vi "Read_Wavedump_Files.vi"(11 "PMTs":string[](array[string])) -> (1 "Plotted data":i32[][][](array[numeric]), 3 "Time Elapsed (s)":u32)   [LabVIEW 2018]
panel:
  in  "Test":string(combo)
  in  "Stop":bool
  in  "?":T1(tab)
  out "Waveform Graph":cluster{"Trace":i32[]}[](graph)
  in  "Viewing Rate (Trace/s)":u32=1 min=1
  in  "Start":bool
  out "Scroll Graph":i32[](graph)
  out "End of file":bool
  in  "Trace":i64
  in  "PMT Number":string
  in  "Close":bool
  # "Plotted data as 3D array"
  # "Channel"
  # "Trace"
  # "Sample"
  # "This vi is used to view previously tested PMTs at a rate of one trace per second for the length of time of recording. PMTs being tested will be viewed using the GNU plot pop up window.\n\nAuto Viewing Tab:\n\nUsed to view waveforms recorded by automattically scrolling through the data at a rate of one recorded waveform in 10000 for the 10 KHz tests (1 in 1000 for files used to develop)\n\nTo view up to 8 PMTs (one electrical tests worth), please enter the test type and the PMT numbers. Then enter the rate at which traces are viewed per second.\n\nPress \"Start\" to start viewing.\n\nUse the tick boxes to change the plots visible. The plots are in the same order the PMT numbers are entered in.\n\nPress \"STOP\" to stop viewing the files.\n\nManual Viewing Tab:\n\nUsed to manually scroll through waveforms one at a  time.\n\nEnter test and PMT number, before selecting which trace to view.\n\nA light indicates if the end of the file has been reached.\n\nPlease note, if the Auto Viewing is running, the Manual Viewing will not work. Please stop this to use the Manual Viewing tab.\n\n\n\n\nPress \"CLOSE\" to close the application."
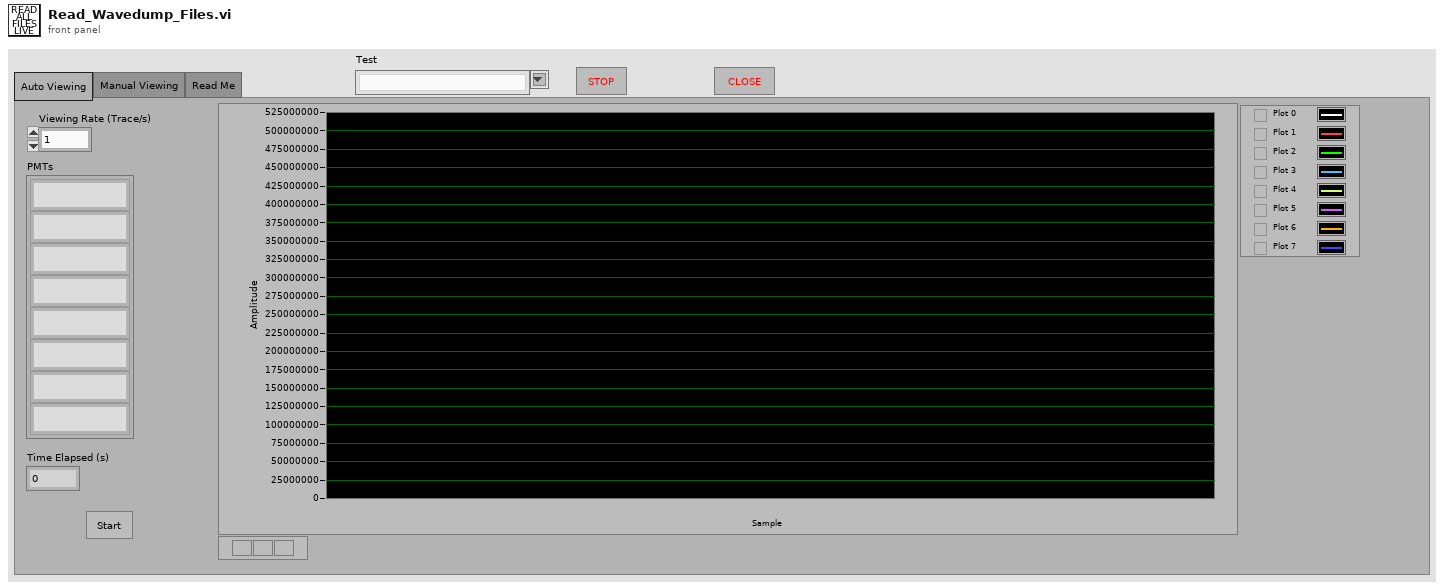
[diagram p1: front panel]
types:
  T1 = enum32{"Auto Viewing", "Manual Viewing", "Read Me"}
  T2 = enum16{"big-endian, network order", "native, host order", "little-endian"}
  T3 = enum16{"open", "replace", "create", "open or create", "replace or create", "replace or create with confirmation"}
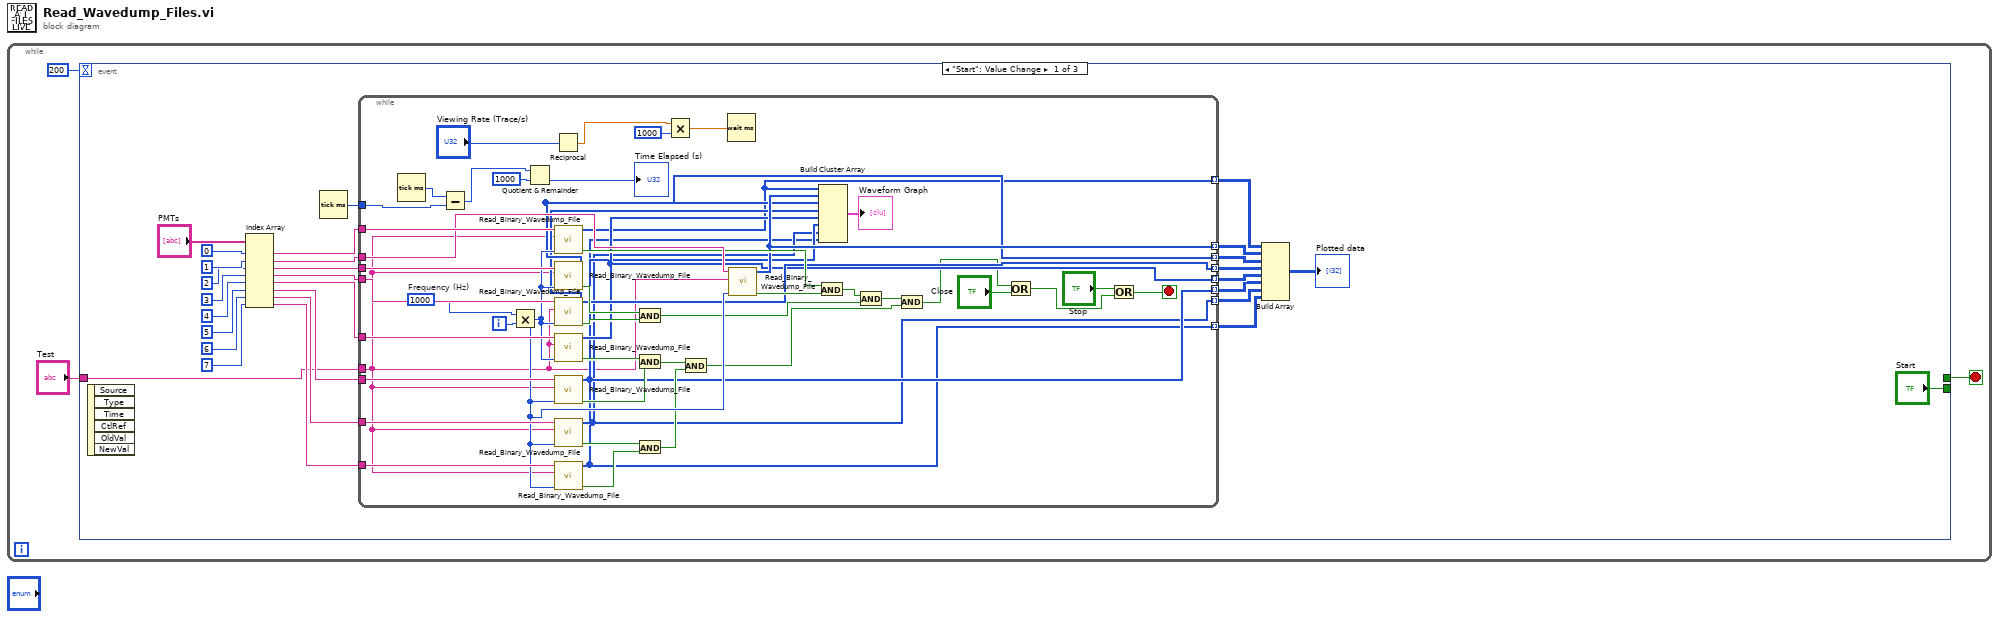
[diagram p0: block diagram]
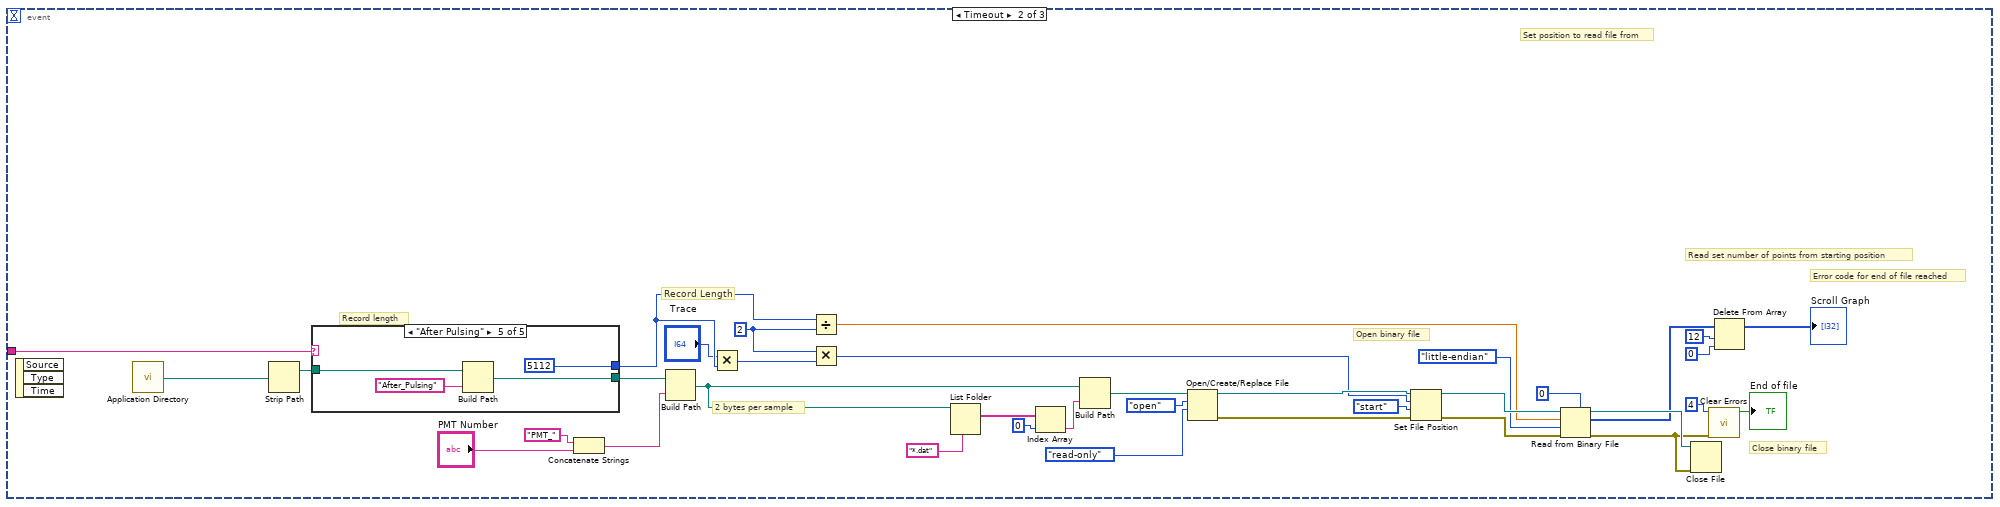
[diagram p2: hidden frame]
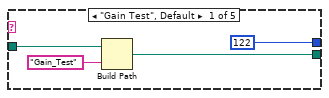
[diagram p3: hidden frame]
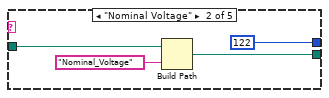
[diagram p4: hidden frame]
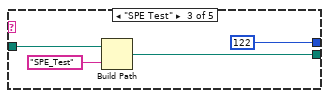
[diagram p5: hidden frame]
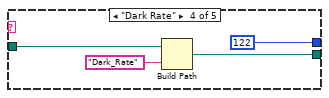
[diagram p6: hidden frame]
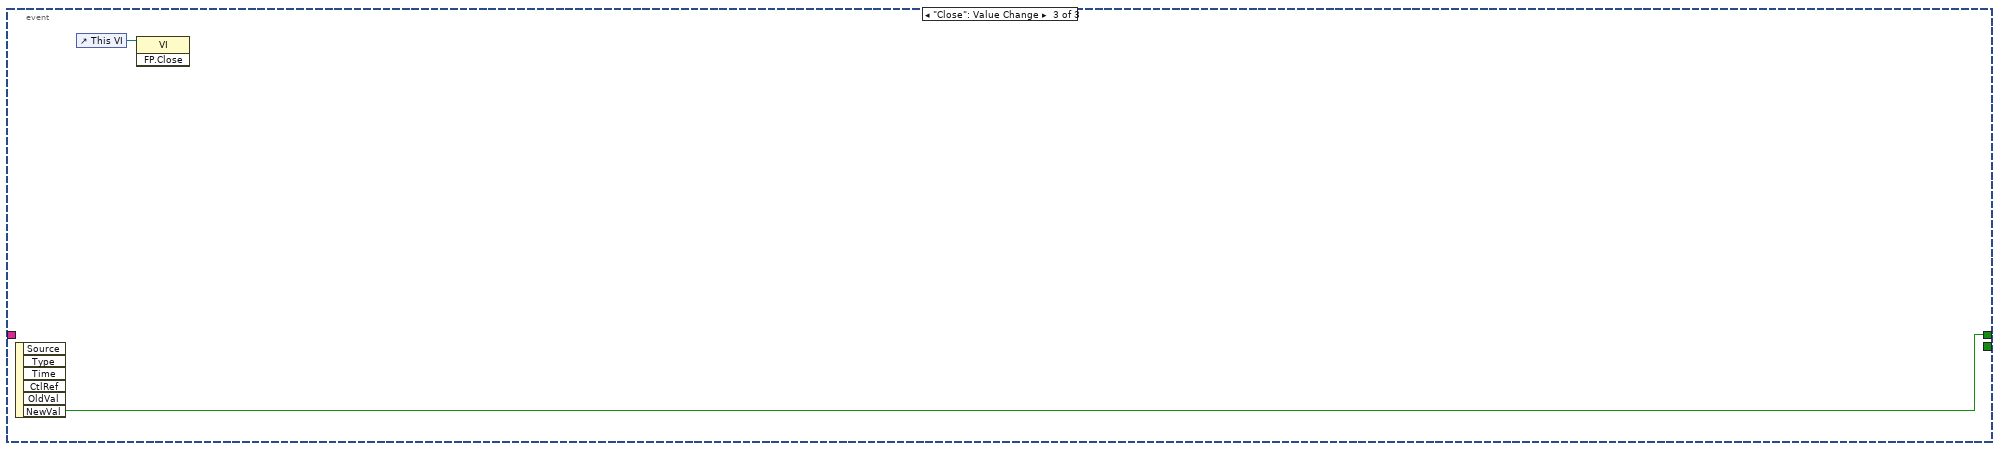
[diagram p7: hidden frame]
diagram:
  n1 = while {
    stop <- w3 stop-if-true
    n2 = event shown="[0] \"Start\": Value Change" {
      selector: _ -> [_ _ _]
      dyn-events: _ -> [_ _ _]
      timeout: 200 -> [_ _ _]
      tunnel: [_ _ w139] -> w3
      tunnel: ["Start" _ _] -> _
      tunnel: "Test" -> [w4 w83 _]
      event "Start": Value Change {
        n3 = event-data() -> ()  [unwired: 1 in, 6 out]
        n4 = Index Array(array="PMTs", index #1=0 ("index"), index #2=1 ("index"), index #3=2 ("index"), index #4=3 ("index"), index #5=4 ("index"), index #6=5 ("index"), index #7=6 ("index"), index #8=7 ("index")) -> (element #1=w24:string, element #2=w23:string, element #3=w22:string, element #4=w21:string, element #5=w20:string, element #6=w19:string, element #7=w18:string, element #8=w17:string)
        n5 = Tick Count (ms)() -> (millisecond timer value=w16:u32)
        n6 = while {
          tunnel: w24 -> [w81]
          tunnel: w23 -> [w80]
          tunnel: w22 -> [w79]
          tunnel: w21 -> [w78]
          tunnel: w20 -> [w77]
          tunnel: w19 -> [w76]
          tunnel: w18 -> [w75]
          tunnel: w17 -> [w74]
          tunnel: w4 -> [w40]
          tunnel: w16 -> [w67]
          tunnel: [w39] -> w15 mode=indexing
          tunnel: [w52] -> w14 mode=indexing
          tunnel: [w51] -> w13 mode=indexing
          tunnel: [w50] -> w12 mode=indexing
          tunnel: [w49] -> w11 mode=indexing
          tunnel: [w48] -> w10 mode=indexing
          tunnel: [w47] -> w9 mode=indexing
          tunnel: [w46] -> w8 mode=indexing
          i -> [w73]
          stop <- w41 stop-if-true
          w72 = 1000  # Frequency (Hz)
          n7 = Tick Count (ms)() -> (millisecond timer value=w68:u32)
          n8 = Subtract(x=w68, y=w67) -> (x-y=w69:u32)
          n9 = Multiply(x=w72, y=w73) -> (x*y=w71:i32)
          n10 = Quotient & Remainder(x=w69, y=u32 1000) -> (floor(x/y)=→"Time Elapsed (s)":u32)  [unwired: 1 out]
          n11 = Reciprocal(x="Viewing Rate (Trace/s)") -> (1/x=w35:dbl)
          n12 = call "Read_Binary_Wavedump_File.vi"("Trace"=w71, "Test"=w40, "PMT Number"=w81) -> ("End of file"=w66:bool, "Trace"=w39:i32[])  [unwired: 6 in]
          n13 = call "Read_Binary_Wavedump_File.vi"("Trace"=w71, "Test"=w40, "PMT Number"=w79) -> ("End of file"=w64:bool, "Trace"=w51:i32[])  [unwired: 6 in]
          n14 = call "Read_Binary_Wavedump_File.vi"("Trace"=w71, "Test"=w40, "PMT Number"=w78) -> ("End of file"=w63:bool, "Trace"=w50:i32[])  [unwired: 6 in]
          n15 = call "Read_Binary_Wavedump_File.vi"("Trace"=w71, "Test"=w40, "PMT Number"=w77) -> ("End of file"=w62:bool, "Trace"=w49:i32[])  [unwired: 6 in]
          n16 = call "Read_Binary_Wavedump_File.vi"("Trace"=w71, "Test"=w40, "PMT Number"=w76) -> ("End of file"=w61:bool, "Trace"=w48:i32[])  [unwired: 6 in]
          n17 = call "Read_Binary_Wavedump_File.vi"("Trace"=w71, "Test"=w40, "PMT Number"=w75) -> ("End of file"=w60:bool, "Trace"=w47:i32[])  [unwired: 6 in]
          n18 = call "Read_Binary_Wavedump_File.vi"("Trace"=w71, "Test"=w40, "PMT Number"=w74) -> ("End of file"=w59:bool, "Trace"=w46:i32[])  [unwired: 6 in]
          n19 = And(x=w64, y=w63) -> (x .and. y?=w56:bool)
          n20 = And(x=w62, y=w61) -> (x .and. y?=w57:bool)
          n21 = And(x=w60, y=w59) -> (x .and. y?=w58:bool)
          n22 = Multiply(x=w35, y=u32 1000 ("milliseconds to wait")) -> (x*y=w36:dbl)
          n23 = And(x=w57, y=w58) -> (x .and. y?=w53:bool)
          n24 = Wait (ms)(milliseconds to wait=w36) -> ()  [unwired: 1 out]
          n25 = call "Read_Binary_Wavedump_File.vi"("Trace"=w71, "Test"=w40, "PMT Number"=w80) -> ("End of file"=w65:bool, "Trace"=w52:i32[])  [unwired: 6 in]
          n26 = And(x=w66, y=w65) -> (x .and. y?=w55:bool)
          n27 = Build Cluster Array(w39, w52, w51, w50, w49, w48, w47, w46) -> (→"Waveform Graph":cluster{"Trace":i32[]}[])
          n28 = And(x=w55, y=w56) -> (x .and. y?=w54:bool)
          n29 = And(x=w54, y=w53) -> (x .and. y?=w45:bool)
          n30 = Or(x=w45, y="Close") -> (x .or. y?=w43:bool)
          n31 = Or(x="Stop", y=w43) -> (x .or. y?=w41:bool)
        }
        n32 = Build Array(w15, w14, w13, w12, w11, w10, w9, w8) -> (→"Plotted data":i32[][][])
      }
      event Timeout {
        w91 = i64 2 ("x")
        # "Record length"
        # "Record Length"
        # "2 bytes per sample"
        # "Error code for end of file reached"
        # "Close binary file"
        # "Read set number of points from starting position"
        # "Set position to read file from"
        # "Open binary file"
        n33 = event-data() -> ()  [unwired: 1 in, 3 out]
        n34 = call <vilib>:"Application Directory.vi"() -> ("Application Directory"=w103:path)
        n35 = Strip Path(path=w103) -> (stripped path=w92:path)  [unwired: 1 out]
        n36 = case shown="\"After Pulsing\"" w83 {
          tunnel: [w120 w123 w127 w132 w136] -> w93
          tunnel: w92 -> [w119 w124 w128 w131 w135]
          tunnel: [122 ("Points to Plot") 122 ("Points to Plot") 122 ("Points to Plot") 122 ("Points to Plot") 5112 ("Points to Plot")] -> w90
          frame "Gain Test", Default {
            n37 = Build Path(base path=w119, name or relative path="Gain_Test") -> (appended path=w120:path)
          }
          frame "Nominal Voltage" {
            n38 = Build Path(base path=w124, name or relative path="Nominal_Voltage") -> (appended path=w123:path)
          }
          frame "SPE Test" {
            n39 = Build Path(base path=w128, name or relative path="SPE_Test") -> (appended path=w127:path)
          }
          frame "Dark Rate" {
            n40 = Build Path(base path=w131, name or relative path="Dark_Rate") -> (appended path=w132:path)
          }
          frame "After Pulsing" {
            n41 = Build Path(base path=w135, name or relative path="After_Pulsing") -> (appended path=w136:path)
          }
        }
        n42 = Concatenate Strings("PMT_" ("name or relative path"), "PMT Number") -> (w101:string)
        n43 = Build Path(base path=w93, name or relative path=w101) -> (appended path=w96:path)
        n44 = Multiply(x="Trace", y=w90) -> (x*y=w88:i64)
        n45 = Divide(x=w90, y=w91) -> (x/y=w104:dbl)
        n46 = Multiply(x=w91, y=w88) -> (x*y=w105:i64)
        n47 = List Folder(path=w96, pattern="*.dat") -> (filenames=w98:string[])  [unwired: 2 in, 3 out]
        n48 = Index Array(array=w98, index=0) -> (element=w95:string)
        n49 = Build Path(base path=w96, name or relative path=w95) -> (appended path=w94:path)
        n50 = Open/Create/Replace File(file path (use dialog)=w94, operation (0:open)=T3."open", access (0:read/write)=enum16{"read/write", "read-only", "write-only"}."read-only") -> (refnum out=w112:refnum<file>, error out=w115:errorcluster)  [unwired: 3 in, 1 out]
        n51 = Set File Position(offset (in bytes) (0)=w105, refnum=w112, from (0:start)=enum16{"start", "end", "current"}."start", error in=w115) -> (refnum out=w111:refnum<file>, error out=w116:errorcluster)
        n52 = Read from Binary File(5:0, 8:w116, 9:T2."little-endian" ("byte order (0:big-endian, network order)"), 10:w104, 11:w111) -> (0:w82:errorcluster, 2:w87:i32[], 3:w110:refnum<file>)  [unwired: 1 in, 1 out]
        n53 = Close File(refnum=w110, error in=w82) -> ()  [unwired: 2 out]
        n54 = call <vilib>:"Clear Errors.vi"("error in (no error)"=w82, "specific error code to clear (0: all)"=4) -> ("specific error cleared?"=→"End of file":bool)  [unwired: 4 in, 1 out]
        n55 = Delete From Array(array=w87, length=12, index=0) -> (array with subset deleted=→"Scroll Graph":i32[])  [unwired: 1 out]
      }
      event "Close": Value Change {
        n56 = event-data() -> ("NewVal"=w139:bool)  [unwired: 1 in, 5 out]
        n57 = control-ref of="This VI"() -> (w138:refnum<vi>)
        n58 = invoke class="VI" method="FP.Close"(reference=w138) -> ()  [unwired: 2 in, 3 out]
      }
    }
  }
